vi "detect_circle_gray.vi"() -> ()   [LabVIEW 2020]
uses:
  <vilib>/vision/NI_Vision_Development_Module.lvlib
panel:
  out "Fitted Circle":T1 {"Average SNR (dB)" format="%.2f"; "Average Strength" format="%.2f"; "Roundness (Real-World)" format="%.2f"; "Radius (Real-World)" format="%.2f"; "Center (Real-World)"."Y" format="%.2f"; "Center (Real-World)"."X" format="%.2f"; "Radius (Pixels)" format="%.2f"; "Center (Pixels)"."Y" format="%.2f"; "Center (Pixels)"."X" format="%.2f"}
  out "Circle Found":bool
  out "Image Out 2":T2(plugin-control)
  in  "error in":errorcluster
  out "Circles (Shape Detection 1)":T3(array[cluster]) {"Position"."Y" format="%.2f"; "Position"."X" format="%.2f"}
  out "error out":errorcluster
  in  "File Path":path
  out "Image Out":T2(plugin-control)
  out "Number of Matches Returned":i32
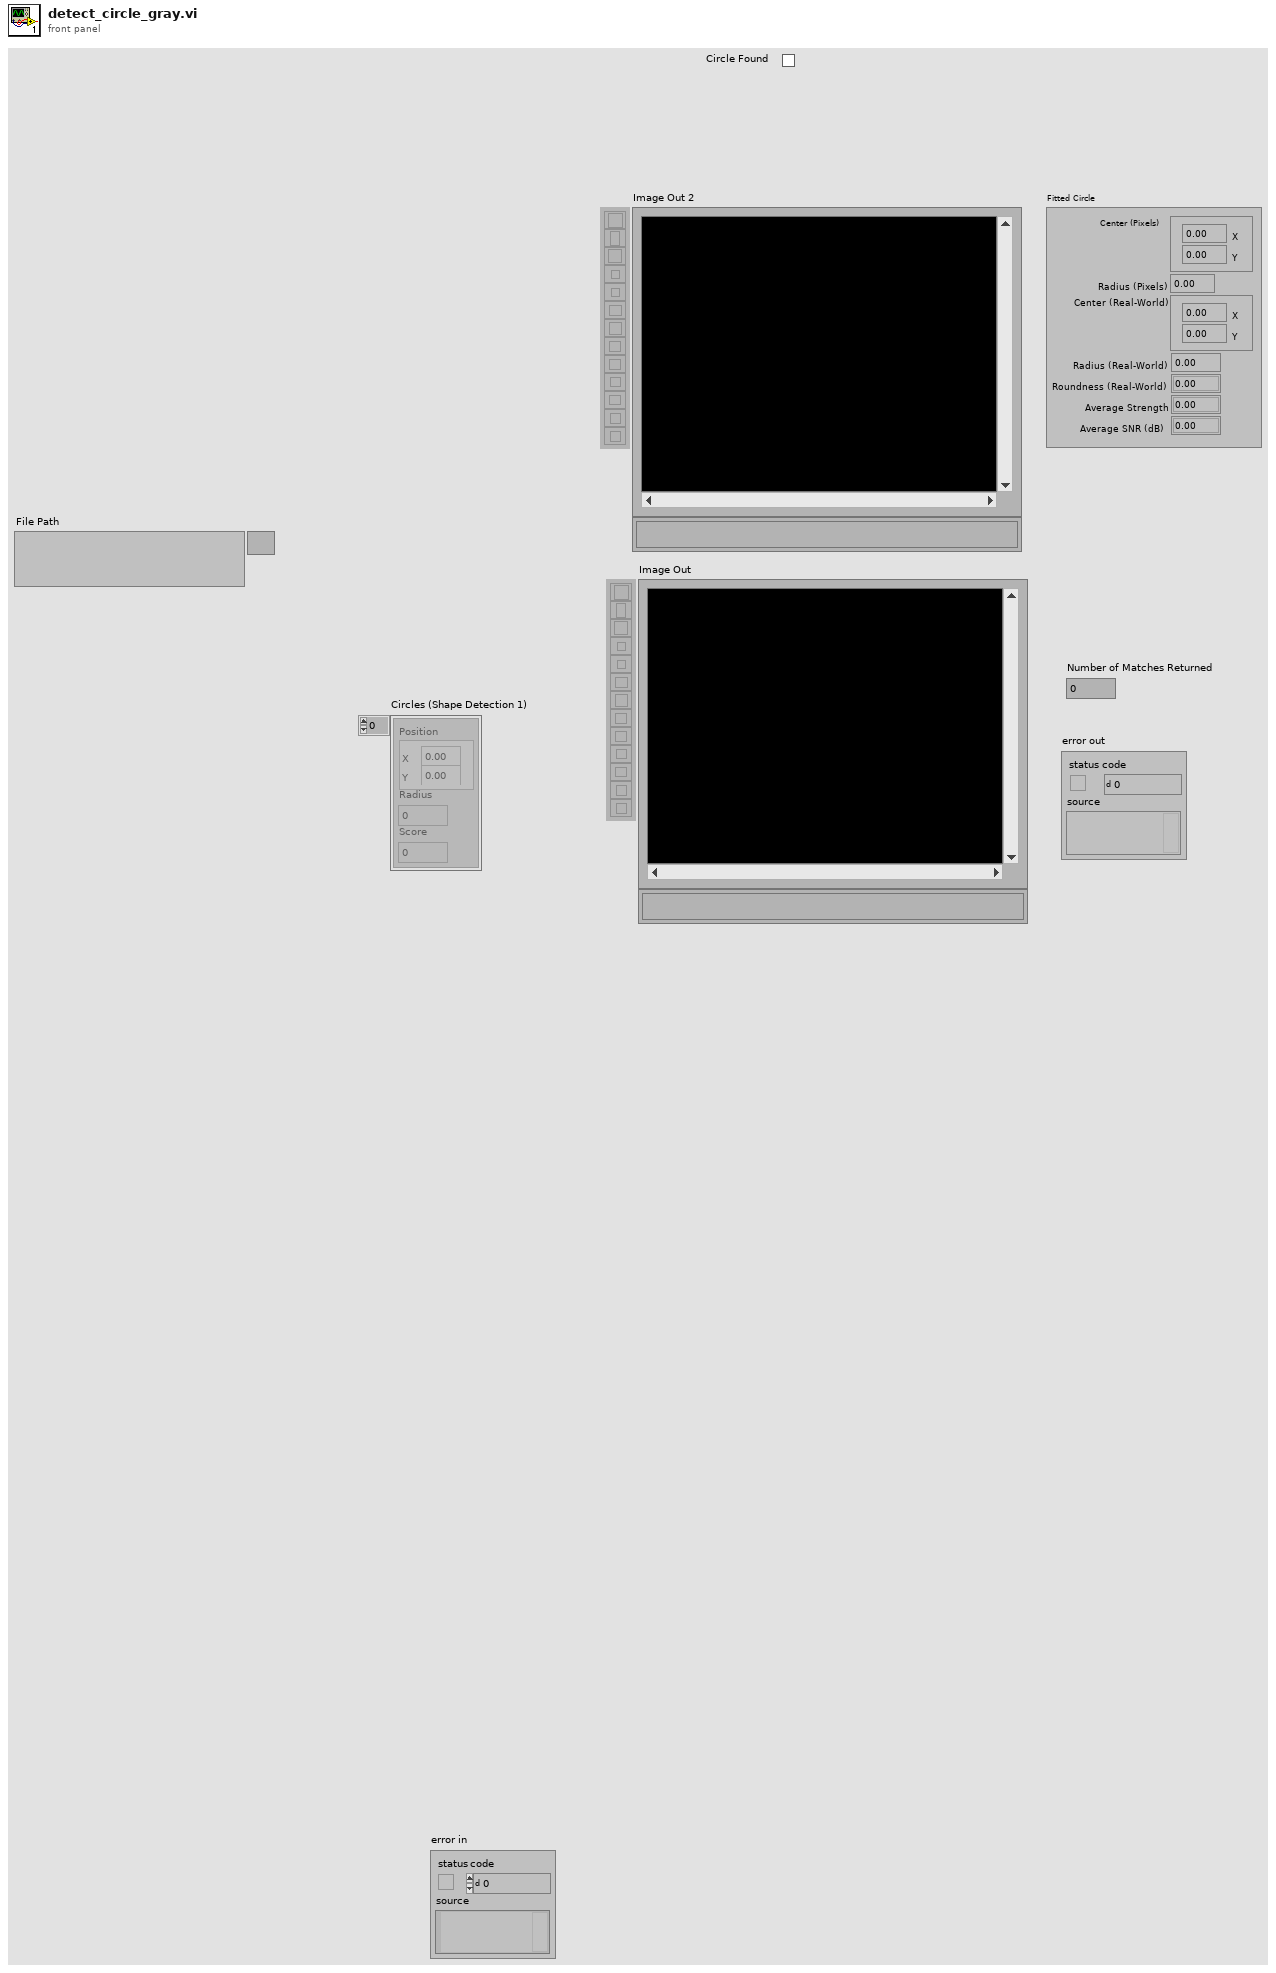
[diagram p1: front panel]
types:
  T1 = cluster{"Center (Pixels)":cluster{"X":sgl, "Y":sgl}, "Radius (Pixels)":dbl, "Center (Real-World)":cluster{"X":sgl, "Y":sgl}, "Radius (Real-World)":dbl, "Roundness (Real-World)":dbl, "Average Strength":dbl, "Average SNR (dB)":dbl}
  T2 = typedef "IMAQ Image.ctl" = refnum<image>
  T3 = cluster{"Position":cluster{"X":sgl, "Y":sgl}, "Radius":dbl, "Score":dbl}[]
  T4 = cluster{"Global Rectangle":i32[], "Contours":cluster{"ID":enum32{"External", "Internal"}, "Type":u32, "Coordinates":i32[]}[]}
  T5 = typedef "Image Type" = u32
  T6 = typedef "IMAQ Circle" = cluster{"Center X":i32, "Center Y":i32, "Inner Radius":i32, "Outer Radius":i32, "Start Angle":dbl, "End Angle":dbl}
  T7 = typedef "ROI Descriptor" = cluster{"Global Rectangle":i32[], "Contours":cluster{"ID":enum32{"External", "Internal"}, "Type":u32, "Coordinates":i32[]}[]}
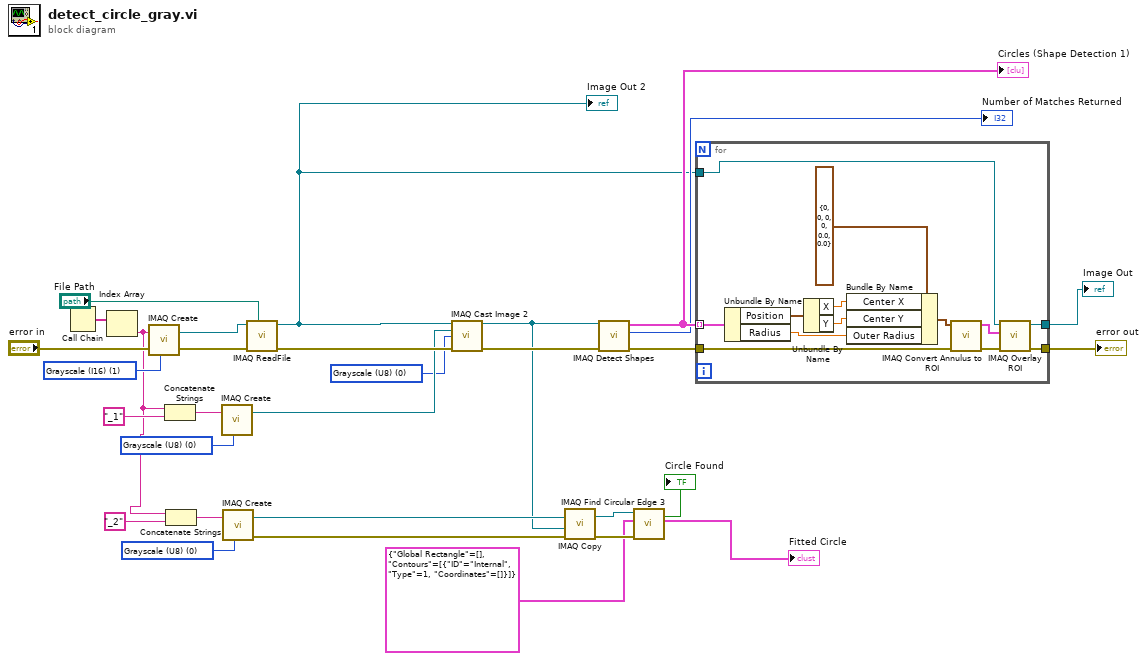
[diagram p0: block diagram]
diagram:
  w12 = T5 0 items=["Grayscale (U8)", "Grayscale (I16)", "Grayscale (SGL)", "Complex (CSG)", "RGB (U32)", "HSL (U32)", "RGB (U64)", "Grayscale (U16)"] ("Image Type")
  w13 = T5 0 items=["Grayscale (U8)", "Grayscale (I16)", "Grayscale (SGL)", "Complex (CSG)", "RGB (U32)", "HSL (U32)", "RGB (U64)", "Grayscale (U16)"] ("Image Type")
  w15 = T5 0 items=["Grayscale (U8)", "Grayscale (I16)", "Grayscale (SGL)", "Complex (CSG)", "RGB (U32)", "HSL (U32)", "RGB (U64)", "Grayscale (U16)"] ("Image Type")
  w27 = T5 1 items=["Grayscale (U8)", "Grayscale (I16)", "Grayscale (SGL)", "Complex (CSG)", "RGB (U32)", "HSL (U32)", "RGB (U64)", "Grayscale (U16)"] ("Image Type")
  n1 = Call Chain() -> (call chain=w28:string[])
  n2 = Index Array(array=w28) -> (element=w9:string)  [unwired: 1 in]
  n3 = call "IMAQ Create"("Image Name"=w9, "Image Type"=w27, "error in (no error)"="error in") -> ("New Image"=w31:T2, "error out"=w30:errorcluster)  [unwired: 1 in, 1 out]
  n4 = Concatenate Strings(w9, "_1" ("string")) -> (w16:string)
  n5 = Concatenate Strings(w9, "_2" ("string")) -> (w11:string)
  n6 = call "IMAQ Create"("Image Name"=w16, "Image Type"=w15) -> ("New Image"=w14:T2)  [unwired: 2 in, 2 out]
  n7 = call "IMAQ Create"("Image Name"=w11, "Image Type"=w12) -> ("New Image"=w7:T2, "error out"=w5:errorcluster)  [unwired: 2 in, 1 out]
  n8 = call "IMAQ ReadFile"("File Path"="File Path", "error in (no error)"=w30, "Image"=w31) -> ("error out"=w20:errorcluster, "Image Out"=w18:T2)  [unwired: 2 in, 5 out]
  "Image Out 2" <- w18
  n9 = call "IMAQ Cast Image 2"("Image Src"=w18, "Image Dst"=w14, "Image Type"=w13, "error in (no error)"=w20) -> ("Image Dst Out"=w6:T2, "error out"=w19:errorcluster)  [unwired: 10 in]
  n10 = call "IMAQ Copy"("error in (no error)"=w5, "Image Dst"=w6, "Image Src"=w7) -> ("error out"=w3:errorcluster, "Image Dst Out"=w4:T2)  [unwired: 3 in]
  n11 = call-poly "IMAQ Detect Shapes"("error in (no error)"=w19, "Image"=w6) -> ("error out"=w22:errorcluster, "Number of Matches Returned"=→"Number of Matches Returned":i32, "Circles"=w26:T3)  [unwired: 5 in, 2 out]
  "Circles (Shape Detection 1)" <- w26
  n12 = call "IMAQ Find Circular Edge 3"("error in (no error)"=w3, "ROI Descriptor"=T4 {"Global Rectangle"=[], "Contours"=[{"ID"=enum."Internal", "Type"=1, "Coordinates"=[]}]}, "Image"=w4) -> ("Fitted Circle"=→"Fitted Circle":T1, "Circle Found"=→"Circle Found":bool)  [unwired: 4 in, 3 out]
  n13 = for {
    tunnel: w26 -> [w38] mode=indexing
    tunnel: w18 -> [w37]
    tunnel: [w36] -> w24
    tunnel: w22 -> [w34]
    tunnel: [w32] -> w21
    n14 = Unbundle By Name(w38) -> ("Position"=w42:cluster{"X":sgl, "Y":sgl}, "Radius"=w39:dbl)
    n15 = Unbundle By Name(w42) -> ("X"=w41:sgl, "Y"=w40:sgl)
    n16 = Bundle By Name(cluster=T6 {"Center X"=0, "Center Y"=0, "Inner Radius"=0, "Outer Radius"=0, "Start Angle"=0.0, "End Angle"=0.0} ("Annulus"), "Center X"=w41, "Center Y"=w40, "Outer Radius"=w39) -> (w44:T6)
    n17 = call "IMAQ Convert Annulus to ROI"("error in (no error)"=w34, "Annulus"=w44) -> ("error out"=w33:errorcluster, "ROI Descriptor"=w35:T7)  [unwired: 7 in]
    n18 = call "IMAQ Overlay ROI"("error in (no error)"=w33, "ROI Descriptor"=w35, "Image"=w37) -> ("error out"=w32:errorcluster, "Image Out"=w36:T2)  [unwired: 7 in]
  }
  "error out" <- w21
  "Image Out" <- w24
